vi "Read log thresholds.vi"(8 "error in (no error)":errorcluster, 11 "Log Producer in":refnum<class "Log Producer.lvclass">) -> (0 "error out":errorcluster, 2 "log thresholds":T1 {"Segment Files By" items=["Time", "Size"]}, 3 "Log Producer out":refnum<class "Log Producer.lvclass">)   [LabVIEW 2020, in "Log Producer.lvclass"]
uses:
  Log Producer.lvclass
  Shared/loggingThreshold_types.ctl
  Log Producer.lvclass/Log Producer.ctl
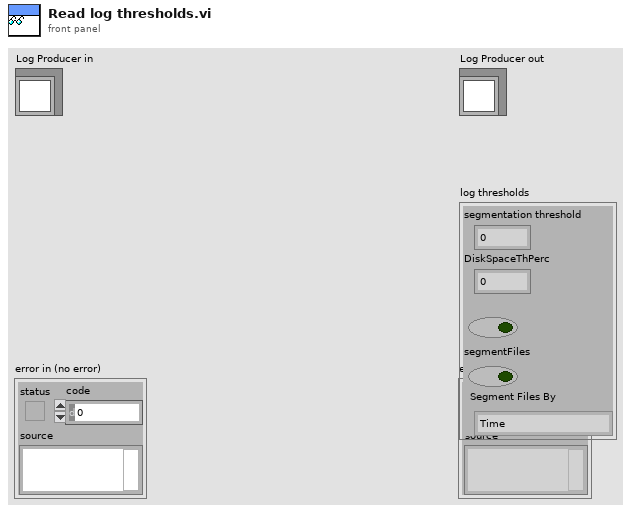
[diagram p1: front panel]
types:
  T1 = typedef "loggingThreshold_types.ctl" = cluster{"segmentation threshold":dbl, "DiskSpaceThPerc":dbl, "checkDiskSpace":bool, "segmentFiles":bool, "Segment Files By":u16}
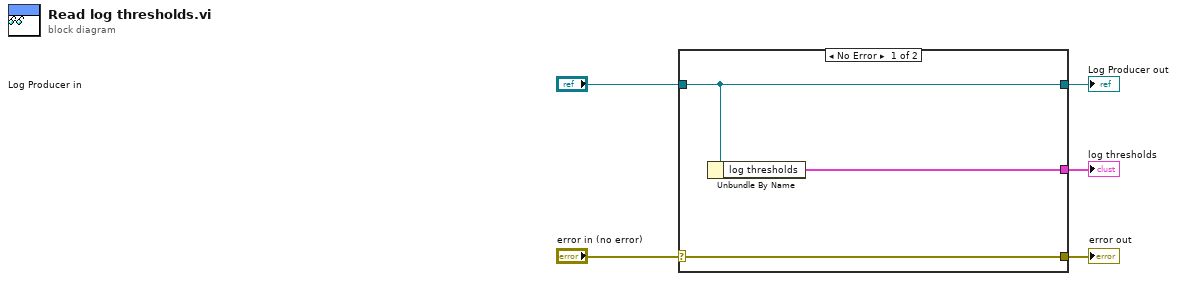
[diagram p0: block diagram]
diagram:
  n1 = case shown="No Error" "error in (no error)" {
    selector: "error in (no error)" -> [w8 w9]
    tunnel: [w8 w9] -> w4
    tunnel: [w7 w10] -> w2
    tunnel: "Log Producer in" -> [w7 w10]
    tunnel: [w6 _] -> w1
    frame No Error {
      n2 = Unbundle By Name(w7) -> ("log thresholds"=w6:T1)
    }
    frame Error {
    }
  }
  "error out" <- w4
  "Log Producer out" <- w2
  "log thresholds" <- w1
